vi "Signal Generator and Filter.vi"(8 "error in (no error)":errorcluster) -> (0 "error out":errorcluster, 2 "Numeric":sgl, 3 "Numeric 2":sgl)   [LabVIEW 2018]
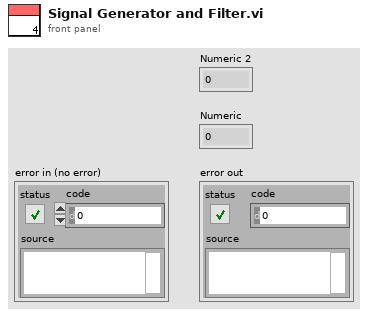
[diagram p1: front panel]
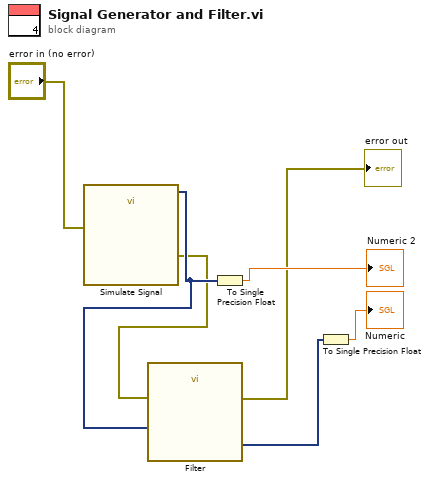
[diagram p0: block diagram]
diagram:
  n1 = call "Simulate Signal"("error in (no error)"="error in (no error)") -> ("Triangle with Gaussian Noise"=w5:dynamicdata, "error out"=w3:errorcluster)  [unwired: 13 in]
  n2 = call "Filter"("error in (no error)"=w3, "Signal"=w5) -> ("error out"=→"error out":errorcluster, "Filtered Signal"=w6:dynamicdata)  [unwired: 8 in]
  n3 = To Single Precision Float(number=w5) -> (single precision float=→"Numeric 2":sgl)
  n4 = To Single Precision Float(number=w6) -> (single precision float=→"Numeric":sgl)
